vi "boxcar_rolling_mean.vi"(8 "window_width_odd":i32=3, 11 "array_in":dbl[](array[numeric])) -> (0 "error out":errorcluster, 1 "length":i32, 2 "first_idx":i32, 3 "array_out":dbl[](array[numeric]))   [LabVIEW 2019]
uses:
  <vilib>/ptbypt/NI_PtbyPt.lvlib
panel:
  # "Out"
  # "In"
  # "must be odd"
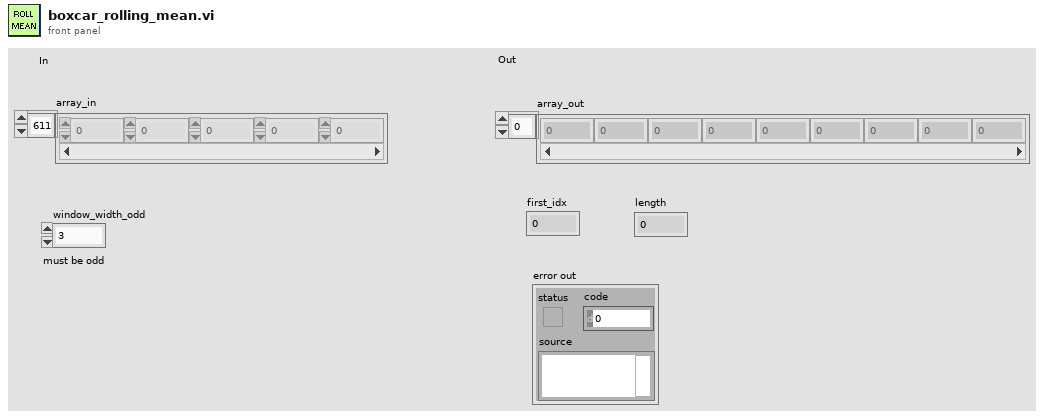
[diagram p1: front panel]
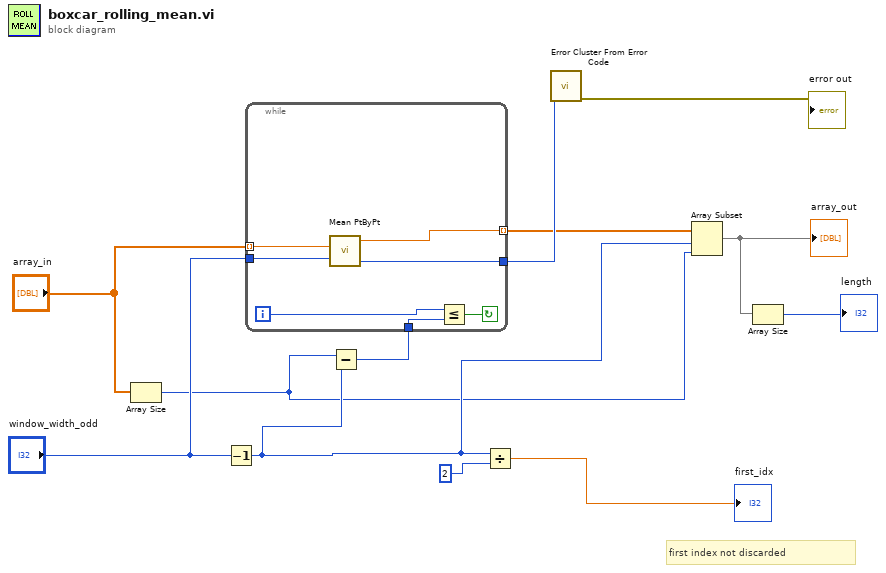
[diagram p0: block diagram]
diagram:
  # "first index not discarded"
  n1 = Array Size(array="array_in") -> (size(s)=w3:i32)
  n2 = Decrement(x="window_width_odd") -> (x-1=w4:i32)
  n3 = Subtract(x=w3, y=w4) -> (x-y=w10:i32)
  n4 = while {
    tunnel: w10 -> [w17]
    tunnel: "array_in" -> [w16] mode=indexing
    tunnel: [w15] -> w5 mode=indexing
    tunnel: [w14] -> w6
    tunnel: "window_width_odd" -> [w13]
    i -> [w19]
    stop <- w18 continue-if-true
    n5 = call <vilib>:"Mean PtByPt.vi"("x"=w16, "sample length"=w13) -> ("mean"=w15:dbl, "error"=w14:i32)  [unwired: 2 in]
    n6 = Less Or Equal?(x=w19, y=w17) -> (x <= y?=w18:bool)
  }
  n7 = Divide(x=w4, y=2) -> (x/y=→"first_idx":dbl)
  n8 = call <vilib>:"Error Cluster From Error Code.vi"("error code (0)"=w6) -> ("error out"=→"error out":errorcluster)  [unwired: 8 in]
  n9 = Array Subset(array=w5, index=w4, length=w3) -> (w2:dbl[])
  "array_out" <- w2
  n10 = Array Size(array=w2) -> (size(s)=→"length":i32)
